vi "com attempt2.vi"() -> ()   [LabVIEW 2020]
uses:
  <vilib>/Instr/_visa.llb/VISA Configure Serial Port (Instr).vi
panel:
  out "Array 2":string[](array[string])
  out "Cluster":cluster{"return":string, "send":string}[](array[cluster])
  out "Array 3":cluster{"send":i32, "return":string}[](array[cluster])
  in  "End Write on Termination Character?":bool=TRUE
  out "Response":string
  in  "Stop":bool
  out "Serial Settings:Number of Bytes at Serial Port":u32
  out "Read 2":bool
  out "Command":string="*IDN?"
  out "Array":i32[](array[numeric]) format="%x"
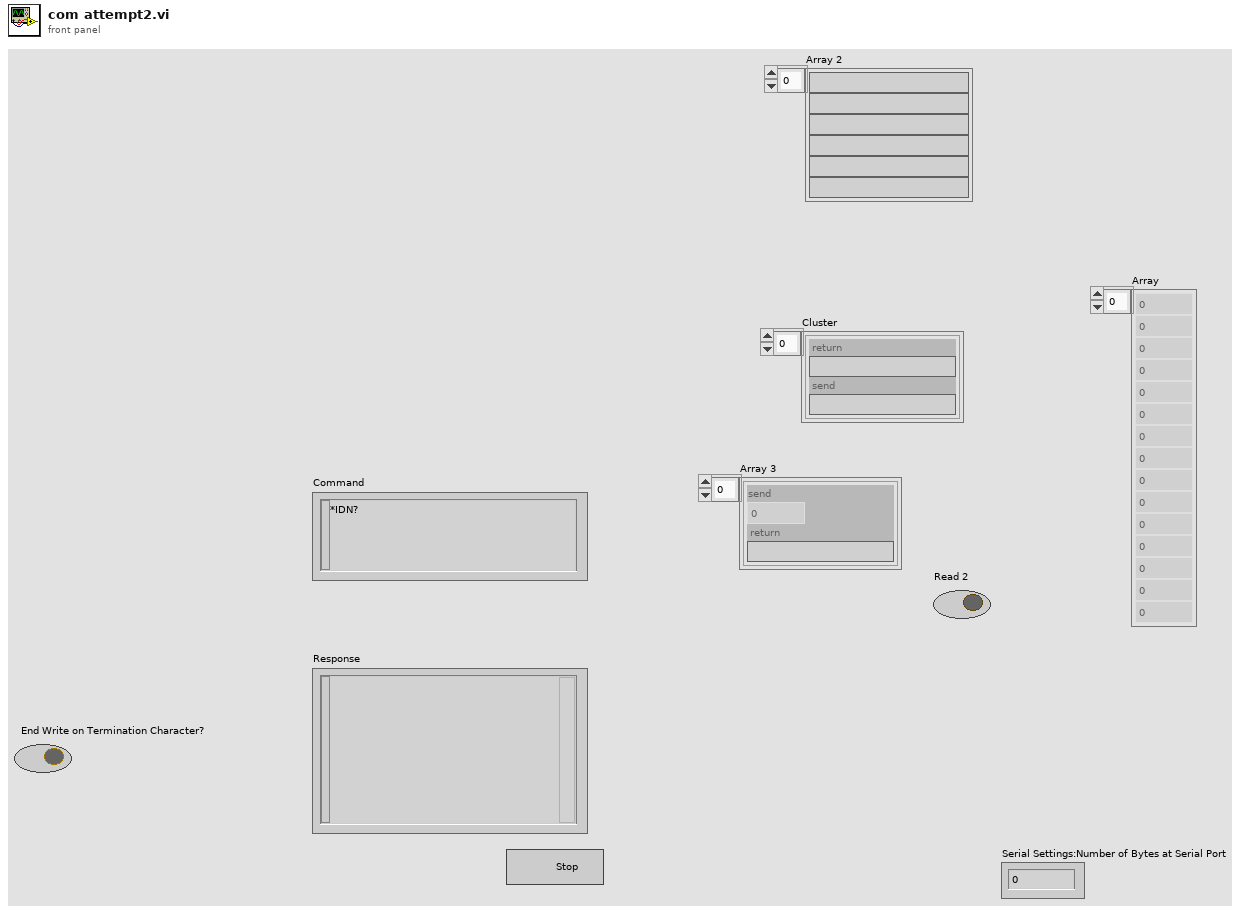
[diagram p1: front panel]
types:
  T1 = cluster{"baud rate":u32, "data bits":u16, "parity":enum16{"None", "Odd", "Even", "Mark", "Space"}, "stop bits":u16, "flow control":u16}
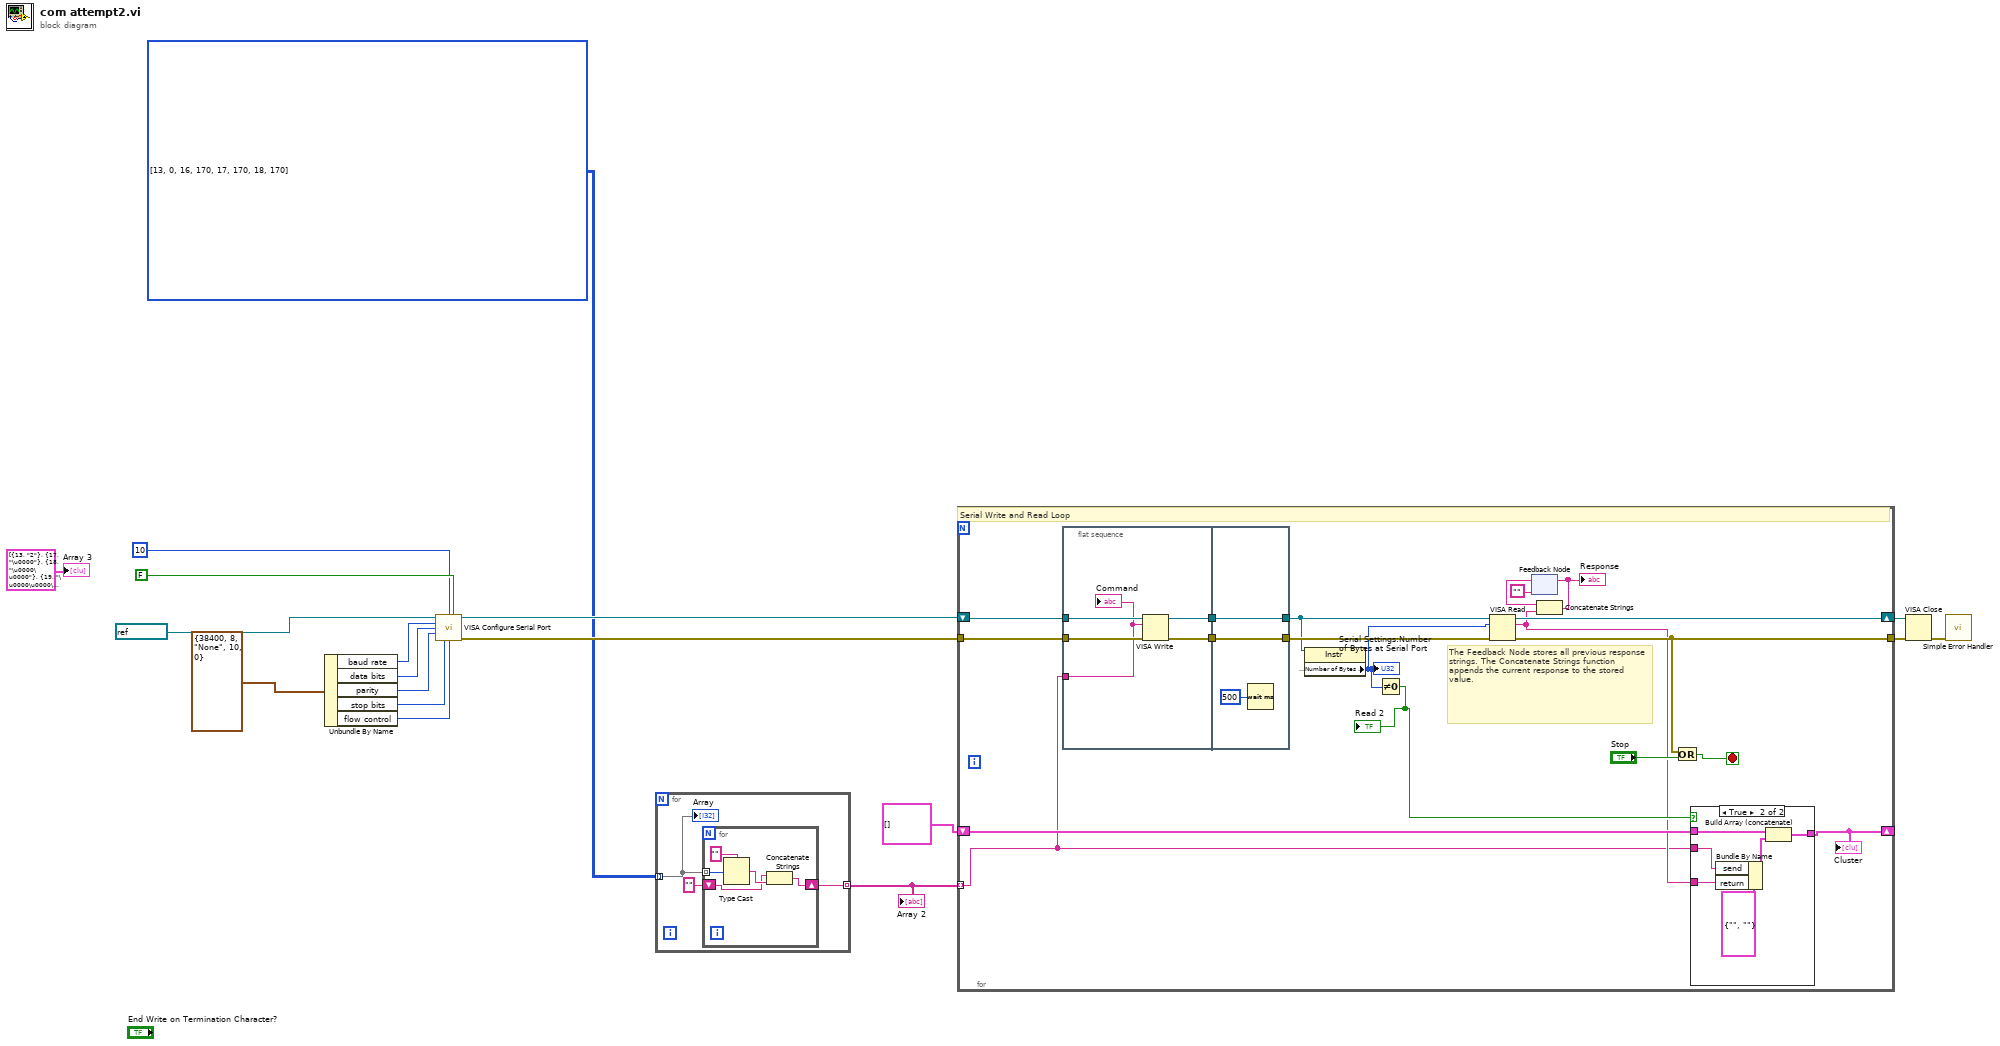
[diagram p0: block diagram]
diagram:
  n1 = Unbundle By Name(T1 {"baud rate"=38400, "data bits"=8, "parity"=enum."None", "stop bits"=10, "flow control"=0} ("Serial Settings")) -> ("baud rate"=w14:u32, "data bits"=w15:u16, "parity"=w16:enum16{"None", "Odd", "Even", "Mark", "Space"}, "stop bits"=w17:u16, "flow control"=w8:u16)
  n2 = call-poly "VISA Configure Serial Port"("VISA resource name"=refnum<visa-resource-name> "COM4", "termination char\n(0xA = '\\n' = LF)"=u8 10 ("Termination Character"), "Enable Termination\nChar (T)"=FALSE ("End Read on Termination Character?"), "baud rate (9600)"=w14, "data bits (8)"=w15, "parity (0:none)"=w16, "stop bits (10: 1 bit)"=w17, "flow control (0:none)"=w8) -> ("VISA resource name out"=w6:refnum<visa-resource-name>, "error out"=w7:errorcluster)  [unwired: 2 in, 4 out]
  n3 = for {
    tunnel: i32[][] [[13, 0], [16, 170], [17, 170], [18, 170]] -> [w21] mode=indexing
    tunnel: [w19] -> w1 mode=indexing
    n4 = for {
      tunnel: w21 -> [w26] mode=indexing
      shift-right: [w23] -> w19
      shift-left: "" -> [w22]
      n5 = Type Cast(type="", x=w26) -> (*(type *) &x=w24:string)
      n6 = Concatenate Strings(w22, w24) -> (w23:string)
    }
    "Array" <- w21
  }
  "Array 2" <- w1
  n7 = for {
    shift-right: [w45] -> w9
    shift-left: w6 -> [w44]
    tunnel: w7 -> [w43]
    tunnel: [w41] -> w10
    shift-right: [w37] -> _
    shift-left: cluster{"return":string, "send":string}[] [] ("Cluster") -> [w35]
    tunnel: w1 -> [w31] mode=indexing
    stop <- w27 stop-if-true
    # "The Feedback Node stores all previous response strings. The Concatenate Strings function appends the current response to the stored value."
    # "Serial Write and Read Loop"
    n8 = flat-sequence {
      tunnel: w44 -> [w57]
      tunnel: w43 -> [w56]
      tunnel: w31 -> [w53]
      tunnel: [w55] -> w39
      tunnel: [w54] -> w38
      tunnel: [w59] -> w42
      tunnel: [w60] -> w34
      tunnel: w39 -> [w60]
      tunnel: w38 -> [w59]
      frame #0 {
        n9 = VISA Write(VISA resource name=w57, write buffer=w53, error in (no error)=w56) -> (VISA resource name out=w55:refnum<visa-resource-name>, error out=w54:errorcluster)  [unwired: 1 out]
        "Command" <- w53
      }
      frame #1 {
        n10 = Wait (ms)(milliseconds to wait=u32 500) -> ()  [unwired: 1 out]
      }
    }
    n11 = property class="Instr"(reference=w34) -> ("Serial Settings:Number of Bytes at Serial Port"=w33:u32)  [unwired: 1 in, 2 out]
    "Serial Settings:Number of Bytes at Serial Port" <- w33
    n12 = Not Equal To 0?(x=w33) -> (x != 0?=w36:bool)
    "Read 2" <- w36
    n13 = VISA Read(VISA resource name=w34, byte count=w33, error in (no error)=w42) -> (VISA resource name out=w45:refnum<visa-resource-name>, read buffer=w32:string, error out=w41:errorcluster)  [unwired: 1 out]
    n14 = feedback #1("") -> (w30:string)
    n15 = Concatenate Strings(w30, w32) -> (w29:string)
    "Response" <- w29
    n16 = feedback-in #1(w29) -> ()
    n17 = Or(x=w41, y="Stop") -> (x .or. y?=w27:bool)
    n18 = case shown="True" w36 {
      tunnel: w31 -> [_ w48]
      tunnel: [w46 w52] -> w37
      tunnel: w35 -> [w46 w51]
      tunnel: w32 -> [_ w47]
      frame False {
      }
      frame True {
        n19 = Bundle By Name(cluster=cluster{"return":string, "send":string} {"return"="", "send"=""} ("Cluster"), "send"=w48, "return"=w47) -> (w49:cluster{"return":string, "send":string})
        n20 = Build Array (concatenate)(w51, w49) -> (w52:cluster{"return":string, "send":string}[])
      }
    }
    "Cluster" <- w37
  }
  n21 = VISA Close(VISA resource name=w9, error in (no error)=w10) -> (error out=w11:errorcluster)
  n22 = call <vilib>:"Simple Error Handler.vi"("error in (no error)"=w11) -> ()  [unwired: 1 in, 8 out]
  "Array 3" <- cluster{"send":i32, "return":string}[] [{"send"=13, "return"="2"}, {"send"=17, "return"="\u0000"}, {"send"=18, "return"="\u0000\u0000"}, {"send"=19, "return"="\u0000\u0000\u0000\u0000"}, {"send"=20, "return"="\u0000\u0000\u0000\u0000\u0000\u0000\u0000\u0000"}] ("Array 3")
